vi "Time.vi"(8 "Reset_Int":dbl, 9 "Configuration":T1(ring), 10 "Reset":bool, 11 "Time_Limit  (ms)":i32) -> (3 "Time_Met":bool)   [LabVIEW 2015]
panel:
  out "Numeric":dbl
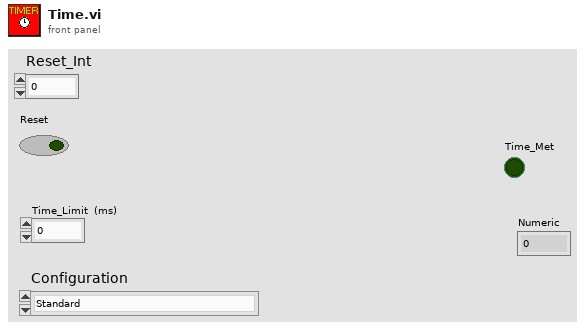
[diagram p1: front panel]
types:
  T1 = enum16{"Standard", "Momentary Falling", "Momentary Rising", "Momentary Falling and Rising"}
  T2 = enum16{"Rising", "Falling", "Falling and Rising"}
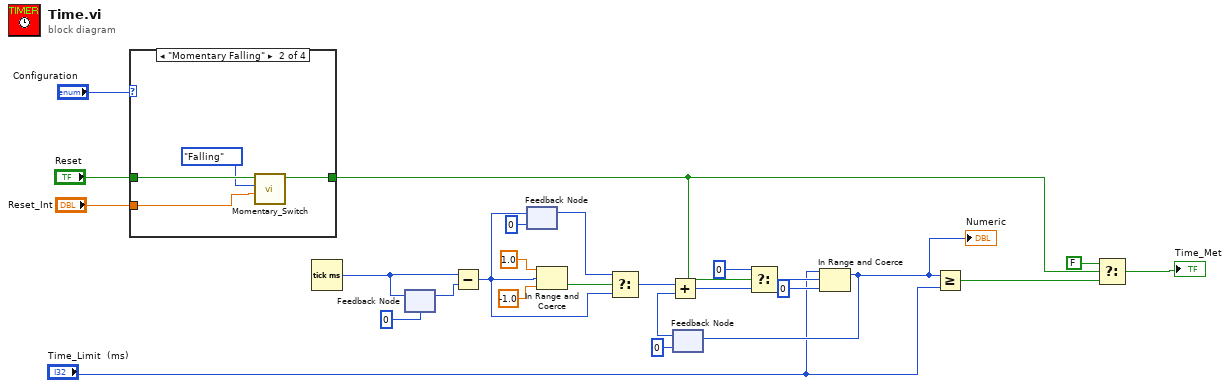
[diagram p0: block diagram]
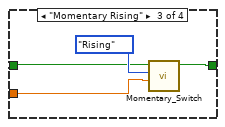
[diagram p3: hidden frame]
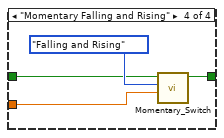
[diagram p4: hidden frame]
diagram:
  n1 = case shown="\"Momentary Falling\"" "Configuration" {
    tunnel: "Reset" -> [w26 w29 w32 w36]
    tunnel: [w26 w30 w33 w38] -> w1
    tunnel: "Reset_Int" -> [_ w27 w31 w35]
    frame "Standard", Default {
    }
    frame "Momentary Falling" {
      n2 = call "Momentary_Switch.vi"("input_int"=w27, "Type"=enum16{"Rising", "Falling"}."Falling" ("Enum"), "input_bol"=w29) -> ("out"=w30:bool)  [unwired: 8 in]
    }
    frame "Momentary Rising" {
      n3 = call "Momentary_Switch.vi"("input_int"=w31, "Type"=enum16{"Rising", "Falling"}."Rising" ("Enum"), "input_bol"=w32) -> ("out"=w33:bool)  [unwired: 8 in]
    }
    frame "Momentary Falling and Rising" {
      n4 = call "Momentary_Switch.vi"("input_int"=w35, "Type"=T2."Falling and Rising" ("Enum"), "input_bol"=w36) -> ("out"=w38:bool)  [unwired: 8 in]
    }
  }
  n5 = Tick Count (ms)() -> (millisecond timer value=w25:u32)
  n6 = feedback #1(u32 0) -> (w24:u32)
  n7 = feedback-in #1(w25) -> ()
  n8 = Subtract(x=w25, y=w24) -> (x-y=w19:u32)
  n9 = feedback #2(u32 0) -> (w20:u32)
  n10 = feedback-in #2(w19) -> ()
  n11 = In Range and Coerce(upper limit=1.0, x=w19, lower limit=-1.0 ("upper limit")) -> (In Range?=w21:bool)  [unwired: 1 out]
  n12 = Select(t=w20, s=w21, f=w19) -> (s? t:f=w18:u32)
  n13 = feedback #3(u32 0) -> (w16:u32)
  n14 = Add(x=w18, y=w16) -> (x+y=w15:u32)
  n15 = Select(t=0, s=w1, f=w15) -> (s? t:f=w10:u32)
  n16 = In Range and Coerce(upper limit="Time_Limit  (ms)", x=w10, lower limit=u32 0) -> (coerced(x)=w9:u32)  [unwired: 1 out]
  "Numeric" <- w9
  n17 = feedback-in #3(w9) -> ()
  n18 = Greater Or Equal?(x=w9, y="Time_Limit  (ms)") -> (x >= y?=w2:bool)
  n19 = Select(t=FALSE, s=w1, f=w2) -> (s? t:f=→"Time_Met":bool)
